vi "Goodness of Fit.vi"(8 "degree of freedom":i32=-1, 9 "Weight":dbl[](array[numeric]), 10 "Best Fit":dbl[](array[numeric]), 11 "Y":dbl[](array[numeric])) -> (0 "error":i32, 1 "RMSE":dbl, 2 "R-square":dbl, 3 "SSE":dbl)   [LabVIEW 2018, in "NI_AALPro.lvlib"]
doc: "Calculates three statistical parameters, <B>SSE</B>, <B>R-square</B>, and <B>RMSE</B>, that describe how well a fitted model matches the original data set."
uses:
  NI_AALPro.lvlib
  <resource>/lvanlys.dll
panel:
  # "goodness of fit"
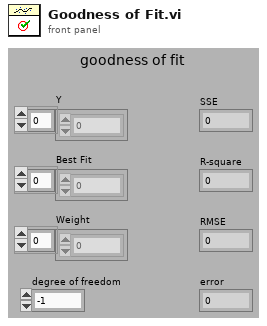
[diagram p1: front panel]
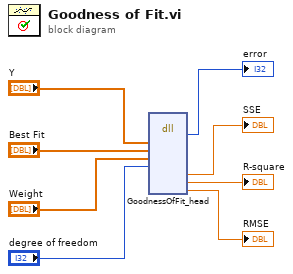
[diagram p0: block diagram]
diagram:
  n1 = dll-call lib="C:/Program Files (x86)/National Instruments/LabVIEW 2018/resource/lvanlys.*" fn="GoodnessOfFit_head"("y"="Y", "bestFit"="Best Fit", "weight"="Weight", "degofFreedom"="degree of freedom") -> (→"error":i32, "SSE"=→"SSE":dbl, "rSquare"=→"R-square":dbl, "RMSE"=→"RMSE":dbl)  [unwired: 10 in, 2 out]
